vi "SetFontFormat.vi"(4 "Size":i32, 5 "列":i32, 6 "斜体":bool, 7 "行":i32, 8 "error":errorcluster caption="错误输入（无错误）", 9 "粗体":bool, 10 "下划线":bool, 11 "Excel._Worksheet":refnum<k7>) -> (0 "error out":errorcluster caption="错误输出", 3 "Excel._Worksheet":refnum<k7>)   [LabVIEW 2014]
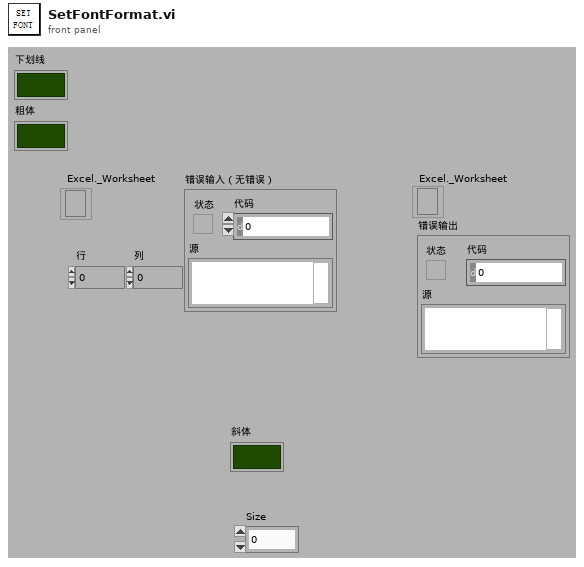
[diagram p1: front panel]
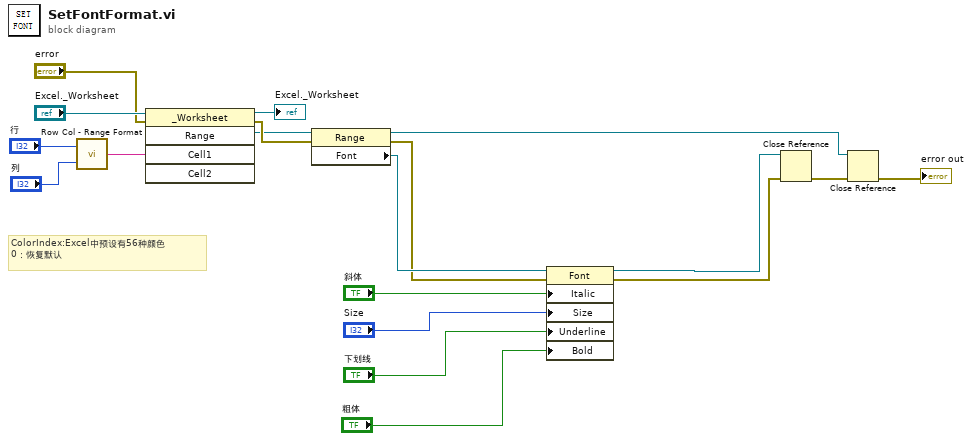
[diagram p0: block diagram]
diagram:
  # "ColorIndex:Excel中预设有56种颜色\n0：恢复默认"
  n1 = call "Row Col - Range Format.vi"("Column"="列", "Row"="行") -> ("Output String"=w5:string)
  n2 = invoke class="_Worksheet" method="Range"(reference="Excel._Worksheet", error in="error", "Cell1"=w5) -> (reference out=→"Excel._Worksheet":refnum<k7>, error out=w15:errorcluster, "Range"=w13:refnum<k7>)  [unwired: 2 in, 2 out]
  n3 = property class="Range"(reference=w13, error in=w15) -> (reference out=w11:refnum<k7>, error out=w7:errorcluster, "Font"=w8:refnum<k7>)
  n4 = property class="Font"(reference=w8, error in=w7, "Italic"="斜体", "Size"="Size", "Underline"="下划线", "Bold"="粗体") -> (reference out=w9:refnum<k7>, error out=w6:errorcluster)
  n5 = Close Reference(reference=w9, error in (no error)=w6) -> (error out=w12:errorcluster)
  n6 = Close Reference(reference=w11, error in (no error)=w12) -> (error out=→"error out":errorcluster)
